vi "ObtainAutoQueue.vi"(0 "VI reference in":refnum<vi> caption="VI reference in (Top-Level)", 11 "Error in":errorcluster caption="Error in (no error)") -> (4 "Queue":refnum<queue>, 15 "Error out":errorcluster)   [LabVIEW 2017, in "VILauncher.lvlib"]
doc: "Obtains the AutoQueue used by the VILauncher toolset. The queue data type is 1D array of variant.\n\nRemember to release the <B>Queue</B> reference when you are done using it. Since this is a named queue you'll need to release the same number of times as you obtain.\n\nThis VI is reentrant, and it doesn't run if there is an error on <B>Error in</B>.\n\nSteen Schmidt\nGPower\n26/12 2012"
uses:
  VILauncher.lvlib
panel:
  # "Copyright © 2013\nSteen Schmidt, GPower\nSee enclosed license file for terms and conditions"
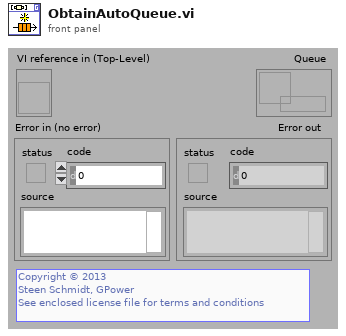
[diagram p1: front panel]
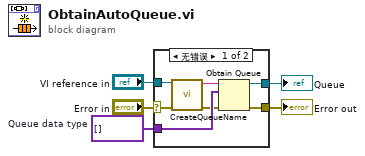
[diagram p0: block diagram]
diagram:
  w2 = variant[] []  # Queue data type
  n1 = case shown="无错误" "Error in" {
    selector: "Error in" -> [w9 w13]
    tunnel: "VI reference in" -> [w6 _]
    tunnel: w2 -> [w12 _]
    tunnel: [w11 _] -> w1
    tunnel: [w10 w13] -> w3
    frame No Error {
      n2 = call "CreateQueueName.vi"("VI reference in"=w6, "Error in"=w9) -> ("Queue name"=w7:string, "Error out"=w8:errorcluster)  [unwired: 12 in]
      n3 = Obtain Queue(name (unnamed)=w7, element data type=w12, error in (no error)=w8) -> (queue out=w11:refnum<queue>, error out=w10:errorcluster)  [unwired: 2 in, 1 out]
    }
    frame Error {
    }
  }
  "Error out" <- w3
  "Queue" <- w1
